vi "Create HSE_v2_Formatter.vi"(6 "Error Line Format Specifier":string="    => Error %1$d: %2$s\n%s", 8 "error in":errorcluster, 9 "Log Line Format Specifier":string="%1$s - %2$-8s - %3$s - %4$s", 10 "Datetime format":string="%.;%Y-%m-%d %H:%M:%S%3u") -> (0 "error out":errorcluster, 3 "HSE_v2_Formatter out":refnum<class "HSE_v2_Formatter.lvclass">)   [LabVIEW 2024, in "hse-logger.lvlib" / "HSE_v2_Formatter.lvclass"]
doc: "Creates a HSE_v2 Formatter object with a default format string and datetime string in ISO format with milliseconds. Errors are displayed in a second line.\n\n<b>Log Line Format Specifier</b> formats the log message in one line.\n------------------------\n 1. Date Time (formatted by the \"Datetime Format\" string)\n 2. Log Level\n 3. Log Message\n 4. Call Chain\n\nIf the Log Record has an active error, <b>Error Line Format Specifier</b> formats the error message in a second line.\n------------------------\n 1. Error Code\n 2. Error Message (cleaned source string)\n 3. Extended error information\n\n____\nHAMPEL SOFTWARE ENGINEERING v2.2.2 (2025-01-16 15:41)"
uses:
  <vilib>/Hampel Software Engineering/HSE Logger/Formatter/HSE_v2_Formatter/HSE_v2_Formatter.lvclass
  <vilib>/Hampel Software Engineering/HSE Logger/Formatter/HSE_v2_Formatter/HSE_v2_Formatter.lvclass/HSE_v2_Formatter.ctl
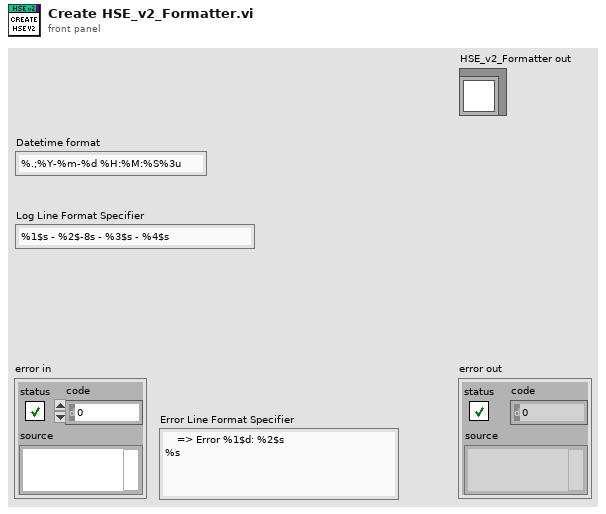
[diagram p1: front panel]
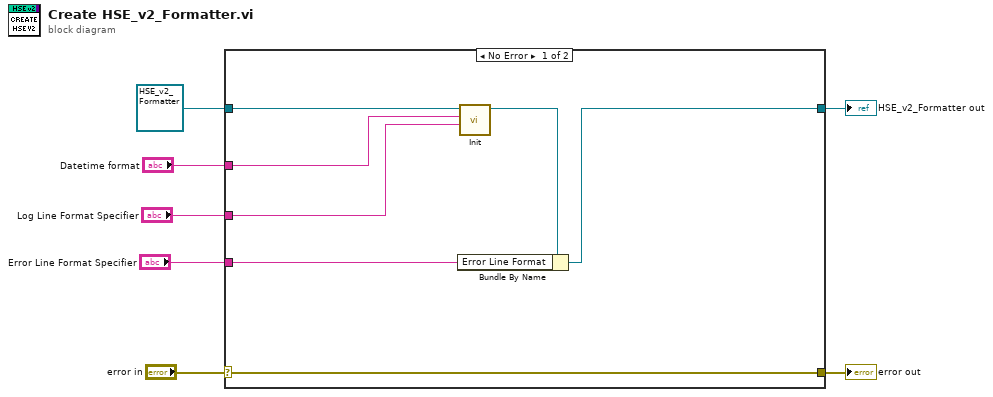
[diagram p0: block diagram]
diagram:
  n1 = case shown="No Error" "error in" {
    selector: "error in" -> [w14 w16]
    tunnel: [w14 w16] -> w6
    tunnel: [w9 w15] -> w4
    tunnel: refnum<class "HSE_v2_Formatter.lvclass"> refnum ("HSE_v2_Formatter in") -> [w13 w15]
    tunnel: "Datetime format" -> [w11 _]
    tunnel: "Log Line Format Specifier" -> [w10 _]
    tunnel: "Error Line Format Specifier" -> [w8 _]
    frame No Error {
      n2 = call-dynamic "Init.vi"("Format Specifier"=w10, "Datetime format"=w11, "Formatter in"=w13) -> ("Formatter out"=w12:refnum<class "HSE_v2_Formatter.lvclass">)  [unwired: 7 in, 1 out]
      n3 = Bundle By Name(cluster=w12, "Error Line Format"=w8) -> (w9:refnum<class "HSE_v2_Formatter.lvclass">)
    }
    frame Error {
    }
  }
  "error out" <- w6
  "HSE_v2_Formatter out" <- w4
